vi "Convert Font To Style Object.vi"(8 "error in (no error)":errorcluster, 10 "Style":T1={"Name"="Calibri", "Font"={"Name"="Calibri", "Size"=12, "Bold"=FALSE, "Italic"=FALSE, "Underline"=18, "Strike"=FALSE, "Color"=0, "Alignment"=1}} {"Font"."Alignment" items=["LEFT"=1, "CENTER"=2, "RIGHT"=3, "BOTH"=4, "MEDIUM_KASHIDA"=5, "DISTRIBUTE"=6, "NUM_TAB"=7, "HIGH_KASHIDA"=8, "LOW_KASHIDA"=9, "THAI_DISTRIBUTE"=10]; "Font"."Underline" items=["Single"=1, "Words"=2, "Double"=3, "Thick"=4, "Dotted"=5, "DottedHeavy"=6, "Dash"=7, "DashedHeavy"=8, "DashLong"=9, "DashLongHeavy"=10, "DotDash"=11, "DashDotHeavy"=12, "DotDotDash"=13, "DashDotDotHeavy"=14, "Wave"=15, "WavyHeavy"=16, "WavyDouble"=17, "None"=18]}) -> (0 "error out":errorcluster, 3 "Style Object":refnum<class "Style.lvclass">)   [LabVIEW 2017, in "Styles.lvlib"]
uses:
  Styles.lvlib
  Style--cluster.ctl
  Font--cluster.ctl
  Underline--ring.ctl
  Alignment--ring.ctl
  Style/Style.lvclass
  Title/Title.lvclass
  C:/Users/Neo/Desktop/Dev_Tools_BR/LabVIEW_NPOI/src/Styles/Style/Style.lvclass
  Heading 1/Heading 1.lvclass
  Heading 2/Heading 2.lvclass
  Heading 3/Heading 3.lvclass
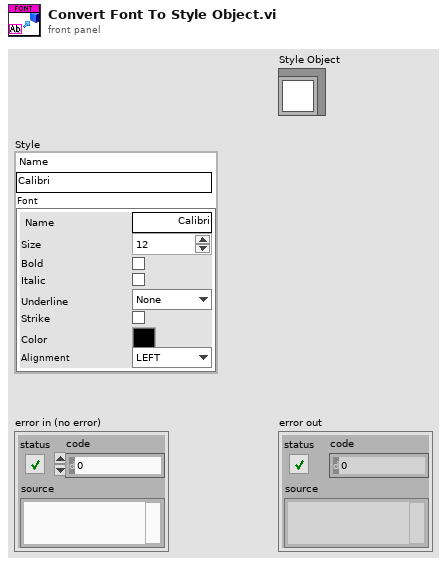
[diagram p1: front panel]
types:
  T1 = typedef "Styles.lvlib/Style--cluster.ctl" = cluster{"Name":string, "Font":T2}
  T2 = typedef "Styles.lvlib/Font--cluster.ctl" = cluster{"Name":string, "Size":i32, "Bold":bool, "Italic":bool, "Underline":T3, "Strike":bool, "Color":u32, "Alignment":T4}
  T3 = typedef "Styles.lvlib/Underline--ring.ctl" = i32
  T4 = typedef "Styles.lvlib/Alignment--ring.ctl" = i32
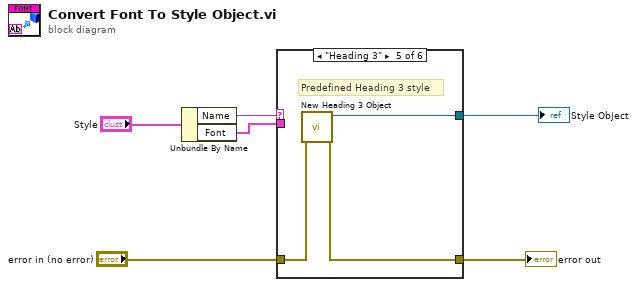
[diagram p0: block diagram]
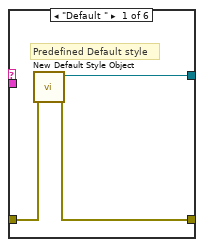
[diagram p2: hidden frame]
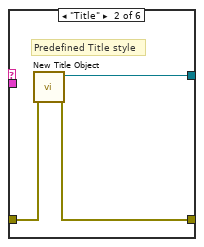
[diagram p3: hidden frame]
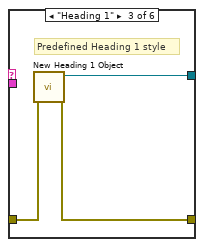
[diagram p4: hidden frame]
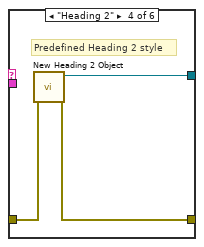
[diagram p5: hidden frame]
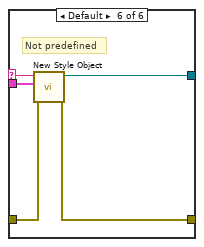
[diagram p6: hidden frame]
diagram:
  n1 = Unbundle By Name("Style") -> ("Name"=w2:string, "Font"=w1:T2)
  n2 = case shown="\"Heading 3\"" w2 {
    selector: w2 -> [_ _ _ _ _ w26]
    tunnel: [w9 w12 w15 w18 w21 w25] -> w6
    tunnel: [w7 w10 w13 w17 w19 w22] -> w5
    tunnel: "error in (no error)" -> [w8 w11 w14 w16 w20 w23]
    tunnel: w1 -> [_ _ _ _ _ w24]
    frame "Default " {
      # "Predefined Default style"
      n3 = call "New Default Style Object.vi"("error in (no error)"=w8) -> ("error out"=w7:errorcluster, "Style out"=w9:refnum<class "Style.lvclass">)  [unwired: 9 in]
    }
    frame "Title" {
      # "Predefined Title style"
      n4 = call "New Title Object.vi"("error in (no error)"=w11) -> ("error out"=w10:errorcluster, "Title out"=w12:refnum<class "Title.lvclass">)  [unwired: 9 in]
    }
    frame "Heading 1" {
      # "Predefined Heading 1 style"
      n5 = call "New Heading 1 Object.vi"("error in (no error)"=w14) -> ("error out"=w13:errorcluster, "Heading 1 out"=w15:refnum<class "Heading 1.lvclass">)  [unwired: 9 in]
    }
    frame "Heading 2" {
      # "Predefined Heading 2 style"
      n6 = call "New Heading 2 Object.vi"("error in (no error)"=w16) -> ("error out"=w17:errorcluster, "Heading 2 out"=w18:refnum<class "Heading 2.lvclass">)  [unwired: 9 in]
    }
    frame "Heading 3" {
      # "Predefined Heading 3 style"
      n7 = call "New Heading 3 Object.vi"("error in (no error)"=w20) -> ("error out"=w19:errorcluster, "Heading 3 out"=w21:refnum<class "Heading 3.lvclass">)  [unwired: 9 in]
    }
    frame Default {
      # "Not predefined"
      # "Not predefined"
      n8 = call "New Style Object.vi"("error in (no error)"=w23, "Font"=w24, "Style Name"=w26) -> ("error out"=w22:errorcluster, "Style out"=w25:refnum<class "Style.lvclass">)  [unwired: 7 in]
    }
  }
  "Style Object" <- w6
  "error out" <- w5
